vi "WriteAttributeOld.vi"(0 "reference in":refnum<class "G#MethodTemplates.lvclass">, 5 "error in (no error)":errorcluster) -> (14 "reference out":refnum<class "G#MethodTemplates.lvclass">, 19 "error out":errorcluster)   [LabVIEW 2020, in "G#MethodTemplates.lvclass"]
uses:
  G#MethodTemplates.lvclass
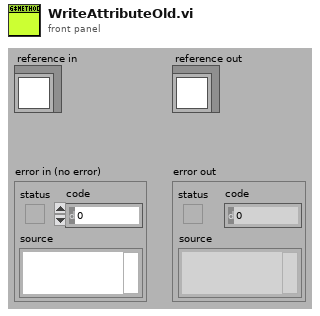
[diagram p1: front panel]
types:
  T1 = typedef "G#MethodTemplates.lvclass/ObjectAttributes.ctl" = cluster{"Numeric":dbl}
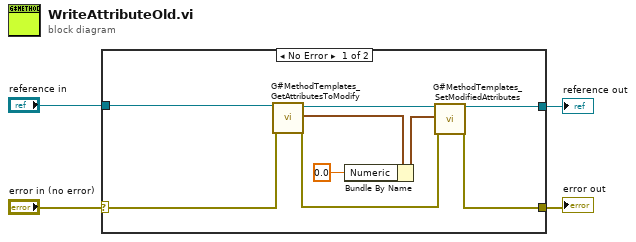
[diagram p0: block diagram]
diagram:
  n1 = case shown="No Error" "error in (no error)" {
    selector: "error in (no error)" -> [w10 w15]
    tunnel: [w12 w15] -> w3
    tunnel: [w9 w14] -> w1
    tunnel: "reference in" -> [w11 w14]
    frame No Error {
      n2 = call "G#MethodTemplates_GetAttributesToModify.vi"("reference in"=w11, "error in (no error)"=w10) -> ("reference out"=w13:refnum<class "G#MethodTemplates.lvclass">, "attributes"=w7:T1, "error out"=w5:errorcluster)  [unwired: 13 in, 2 out]
      n3 = Bundle By Name(cluster=w7, "Numeric"=0.0 ("Attribute1")) -> (w6:T1)
      n4 = call "G#MethodTemplates_SetModifiedAttributes.vi"("reference in"=w13, "attributes"=w6, "error in (no error)"=w5) -> ("reference out"=w9:refnum<class "G#MethodTemplates.lvclass">, "error out"=w12:errorcluster)  [unwired: 15 in]
    }
    frame Error {
    }
  }
  "error out" <- w3
  "reference out" <- w1
